vi "Get Current_Acting_control.vi"(8 "error in (no error)":errorcluster, 11 "Model_Predictor in":refnum<class "Model_Predictor.lvclass">) -> (0 "error out":errorcluster, 2 "current_acting_control":bool, 3 "Model_Predictor out":refnum<class "Model_Predictor.lvclass">)   [LabVIEW 2021, in "MBPOnOff_Controller.lvlib" / "Model_Predictor.lvclass"]
uses:
  Model_Predictor.lvclass
  Model_Predictor.lvclass/Model_Predictor.ctl
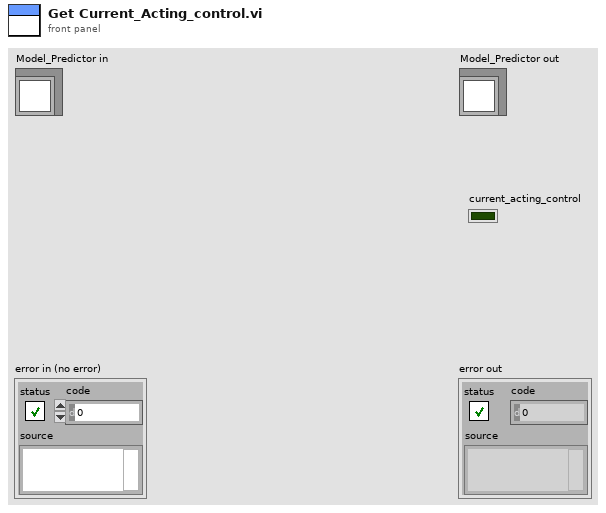
[diagram p1: front panel]
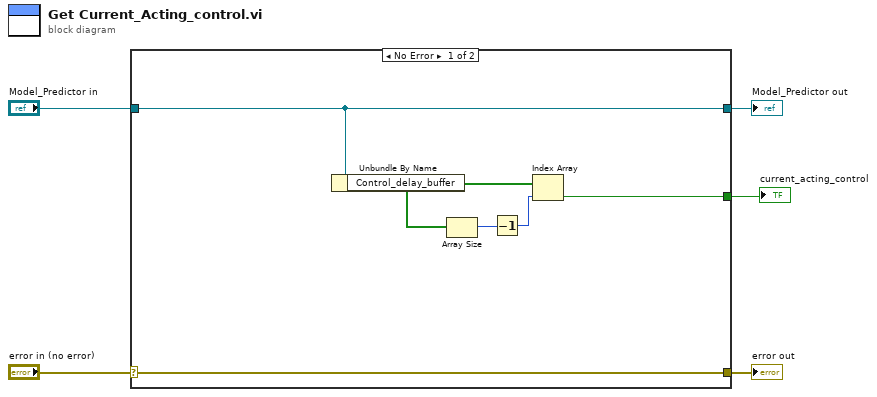
[diagram p0: block diagram]
diagram:
  n1 = case shown="No Error" "error in (no error)" {
    selector: "error in (no error)" -> [w11 w13]
    tunnel: [w11 w13] -> w4
    tunnel: [w10 w12] -> w2
    tunnel: "Model_Predictor in" -> [w10 w12]
    tunnel: [w6 _] -> w1
    frame No Error {
      n2 = Unbundle By Name(w10) -> ("Control_delay_buffer"=w9:bool[])
      n3 = Array Size(array=w9) -> (size(s)=w8:i32)
      n4 = Decrement(x=w8) -> (x-1=w7:i32)
      n5 = Index Array(array=w9, index=w7) -> (element=w6:bool)
    }
    frame Error {
    }
  }
  "error out" <- w4
  "Model_Predictor out" <- w2
  "current_acting_control" <- w1
